vi "SaveBone.vi"(8 "error in (no error)":errorcluster, 11 "Bone Refnum":refnum<k24>) -> (0 "error out":errorcluster, 3 "Bone":T1)   [LabVIEW 2017, in "LeapMotion.lvlib"]
uses:
  LeapMotion.lvlib
  TypeDefs/LEAPbone.ctl
  TypeDefs/LEAPvector.ctl
  C:/Users/snordinh/Desktop/LEAP/LEAP-sign-language-test/LeapMotion/Dynamic Libraries/LeapCSharp.NET4.5.dll
  Dynamic Libraries/LeapCSharp.NET4.5.dll
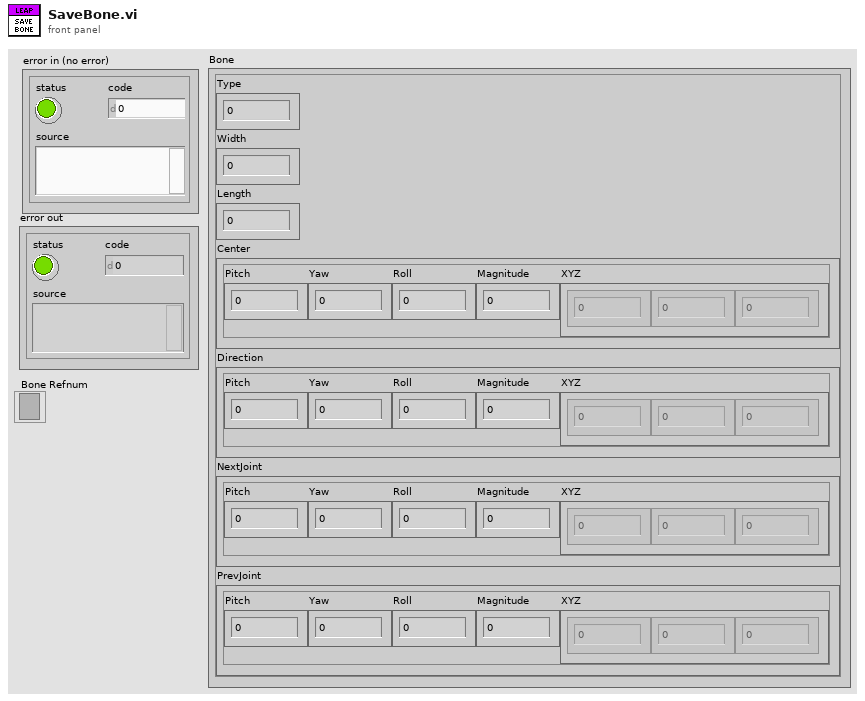
[diagram p1: front panel]
types:
  T1 = typedef "LeapMotion.lvlib/LEAPbone.ctl" = cluster{"Type":i32, "Width":sgl, "Length":sgl, "Center":T2, "Direction":T2, "NextJoint":T2, "PrevJoint":T2}
  T2 = typedef "LeapMotion.lvlib/LEAPvector.ctl" = cluster{"Pitch":sgl, "Yaw":sgl, "Roll":sgl, "Magnitude":sgl, "XYZ":sgl[]}
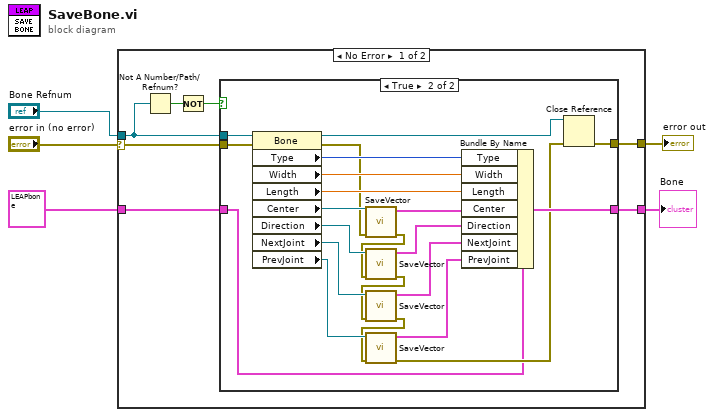
[diagram p0: block diagram]
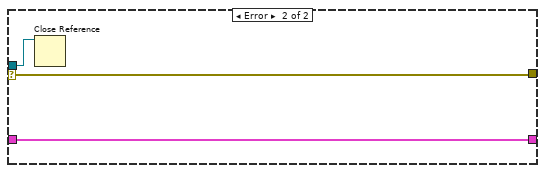
[diagram p3: hidden frame]
diagram:
  n1 = case shown="No Error" "error in (no error)" {
    selector: "error in (no error)" -> [w10 w38]
    tunnel: [w12 w37] -> w5
    tunnel: "Bone Refnum" -> [w9 w39]
    tunnel: [w11 w38] -> w3
    tunnel: T1 {"Type"=0, "Width"=0.0, "Length"=0.0, "Center"={"Pitch"=0.0, "Yaw"=0.0, "Roll"=0.0, "Magnitude"=0.0, "XYZ"=[]}, "Direction"={"Pitch"=0.0, "Yaw"=0.0, "Roll"=0.0, "Magnitude"=0.0, "XYZ"=[]}, "NextJoint"={"Pitch"=0.0, "Yaw"=0.0, "Roll"=0.0, "Magnitude"=0.0, "XYZ"=[]}, "PrevJoint"={"Pitch"=0.0, "Yaw"=0.0, "Roll"=0.0, "Magnitude"=0.0, "XYZ"=[]}} ("Bone") -> [w6 w37]
    frame No Error {
      n2 = Not A Number/Path/Refnum?(number/path/refnum=w9) -> (NaN/Path/Refnum?=w8:bool)
      n3 = Not(x=w8) -> (.not. x?=w7:bool)
      n4 = case shown="True" w7 {
        tunnel: [w13 w36] -> w12
        tunnel: w9 -> [_ w20]
        tunnel: [w14 w18] -> w11
        tunnel: w10 -> [w14 w16]
        tunnel: w6 -> [w13 w15]
        frame False {
        }
        frame True {
          n5 = property class="Bone"(reference=w20, error in=w16) -> (reference out=w19:refnum<k24>, error out=w21:errorcluster, "Type"=w29:i32, "Width"=w30:sgl, "Length"=w31:sgl, "Center"=w28:refnum<k24>, "Direction"=w27:refnum<k24>, "NextJoint"=w26:refnum<k24>, "PrevJoint"=w25:refnum<k24>)
          n6 = call "SaveVector.vi"("error in (no error)"=w21, "Vector Refnum"=w28) -> ("error out"=w22:errorcluster, "LEAPvector"=w32:T2)  [unwired: 8 in]
          n7 = call "SaveVector.vi"("error in (no error)"=w22, "Vector Refnum"=w27) -> ("error out"=w23:errorcluster, "LEAPvector"=w33:T2)  [unwired: 8 in]
          n8 = call "SaveVector.vi"("error in (no error)"=w23, "Vector Refnum"=w26) -> ("error out"=w24:errorcluster, "LEAPvector"=w34:T2)  [unwired: 8 in]
          n9 = call "SaveVector.vi"("error in (no error)"=w24, "Vector Refnum"=w25) -> ("error out"=w17:errorcluster, "LEAPvector"=w35:T2)  [unwired: 8 in]
          n10 = Bundle By Name(cluster=w15, "Type"=w29, "Width"=w30, "Length"=w31, "Center"=w32, "Direction"=w33, "NextJoint"=w34, "PrevJoint"=w35) -> (w36:T1)
          n11 = Close Reference(reference=w19, error in (no error)=w17) -> (error out=w18:errorcluster)
        }
      }
    }
    frame Error {
      n12 = Close Reference(reference=w39) -> ()  [unwired: 1 in, 1 out]
    }
  }
  "Bone" <- w5
  "error out" <- w3
